vi "Define Limit Line.vi"(5 "Connect Point":bool[](array[boolean])=[TRUE], 7 "Amplitude":dbl[](array[numeric])=[-20.0], 8 "error in (no error)":errorcluster, 9 "X Axis":dbl[](array[numeric])=[1000000000.0], 10 "Limit Line (1: Line1)":u16(ring)=1 items=["Line1"=1, "Line2"=2], 11 "VISA resource name":refnum<visa-resource-name>) -> (0 "error out":errorcluster, 3 "VISA resource name out":refnum<visa-resource-name>)   [LabVIEW 2014, in "Agilent ESA PSA Series.lvlib"]
doc: "Configures specified limit line."
uses:
  Agilent ESA PSA Series.lvlib
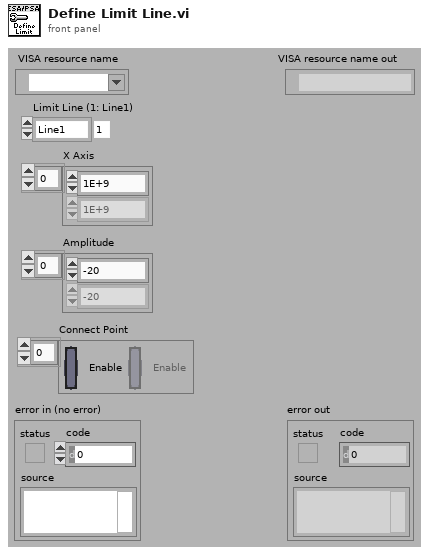
[diagram p1: front panel]
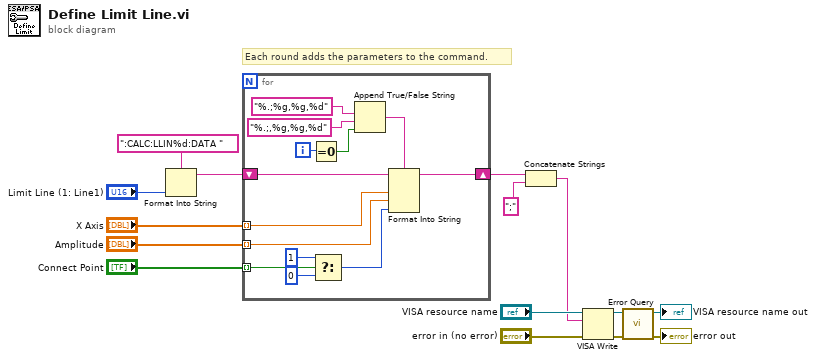
[diagram p0: block diagram]
diagram:
  # "Each round adds the parameters to the command."
  n1 = Format Into String(format string=":CALC:LLIN%d:DATA ", "Limit Line (1: Line1)") -> (resulting string=w8:string)  [unwired: 2 in, 1 out]
  n2 = for {
    shift-right: [w23] -> w3
    shift-left: w8 -> [w22]
    tunnel: "X Axis" -> [w21] mode=indexing
    tunnel: "Amplitude" -> [w20] mode=indexing
    tunnel: "Connect Point" -> [w19] mode=indexing
    i -> [w28]
    n3 = Equal To 0?(x=w28) -> (x = 0?=w27:bool)
    n4 = Select(t=1, s=w19, f=0) -> (s? t:f=w16:i32)
    n5 = Append True/False String(1:w27, 2:"%.;,%g,%g,%d" ("format string"), 3:"%.;%g,%g,%d" ("format string")) -> (0:w24:string)  [unwired: 1 in]
    n6 = Format Into String(format string=w24, initial string=w22, w21, w20, w16) -> (resulting string=w23:string)  [unwired: 1 in, 1 out]
  }
  n7 = Concatenate Strings(w3, ";" ("string")) -> (w2:string)
  n8 = VISA Write(VISA resource name="VISA resource name", write buffer=w2, error in (no error)="error in (no error)") -> (VISA resource name out=w13:refnum<visa-resource-name>, error out=w11:errorcluster)  [unwired: 1 out]
  n9 = call "Error Query.vi"("error in (no error)"=w11, "VISA resource name"=w13) -> ("error out"=→"error out":errorcluster, "VISA resource name out"=→"VISA resource name out":refnum<visa-resource-name>)  [unwired: 6 in, 2 out]
